vi "llh2lcc.vi"(8 "ecef ref":dbl[](array[numeric]) format="%#_19f", 9 "hgt":dbl, 10 "lon":dbl, 11 "lat":dbl) -> (3 "lcc":dbl[](array[numeric]))   [LabVIEW 2015]
uses:
  <vilib>/Analysis/Matrix/Numeric/Conversions/Array To Matrix - RA.vi
  <vilib>/Analysis/Matrix/Numeric/Conversions/Array To Matrix - RA2.vi
  <vilib>/Analysis/Matrix/Numeric/Multiply/Multiply - RM,RM.vi
  <vilib>/Analysis/Matrix/Numeric/Conversions/Matrix To Array - RM.vi
  <vilib>/Analysis/Matrix/NI_Matrix.lvlib
panel:
  out "ecef":dbl[](array[numeric]) format="%#_19f"
  out "DCM(ecef2lcc)":dbl[][](array[numeric])
  out "N":dbl format="%#_19f"
  out "b^2/a^2":dbl
  out "cos(lam)":dbl
  out "sin(lam)":dbl
  out "sin(phi)":dbl
  out "cos(phi)":dbl
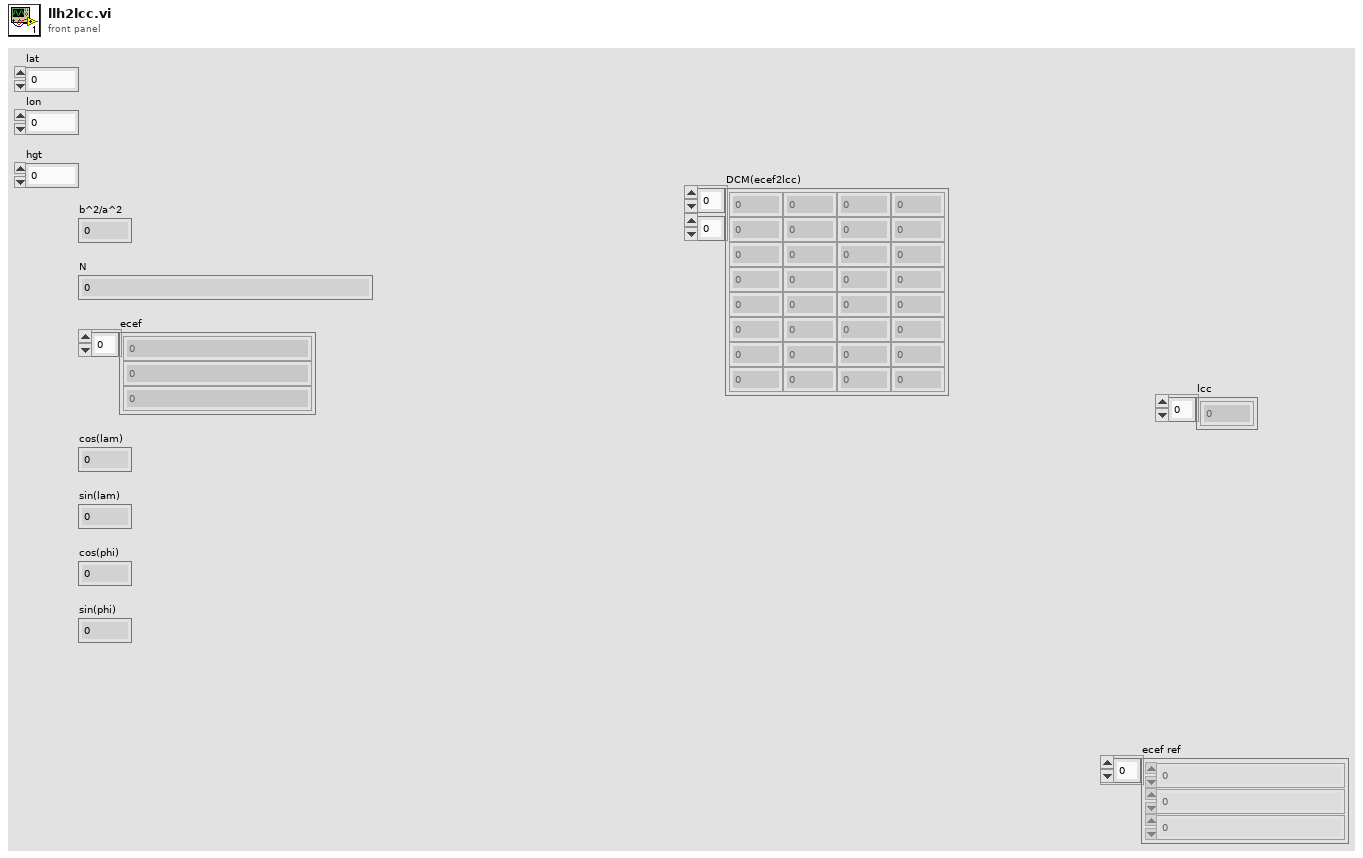
[diagram p1: front panel]
types:
  T1 = typedef "NI_Matrix.lvlib/RealMatrix.ctl" = dbl[][]
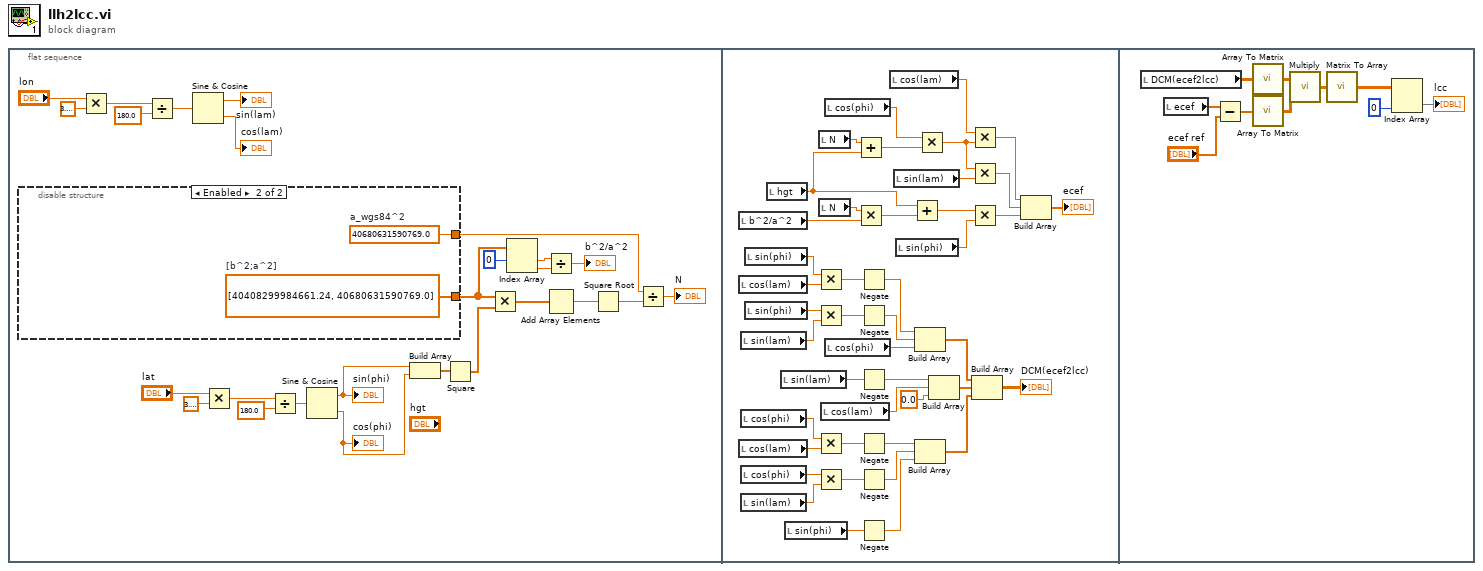
[diagram p0: block diagram]
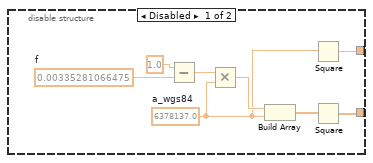
[diagram p2: hidden frame]
diagram:
  n1 = flat-sequence {
    frame #0 {
      n2 = disable-structure shown="Enabled" {
        disable-tunnel: [w29 w36] -> w16
        disable-tunnel: [w27 w35] -> w13
        frame Disabled {
          w34 = 0.00335281066475  # f
          w28 = 6378137.0  # a_wgs84
          n3 = Subtract(x=1.0, y=w34) -> (x-y=w32:dbl)
          n4 = Multiply(x=w32, y=w28) -> (x*y=w31:dbl)
          n5 = Build Array(w31, w28) -> (w30:dbl[])
          n6 = Square(x=w28) -> (x^2=w27:dbl)
          n7 = Square(x=w30) -> (x^2=w29:dbl[])
        }
        frame Enabled {
          w35 = 40680631590769.0  # a_wgs84^2
          w36 = dbl[] [40408299984661.24, 40680631590769.0]  # [b^2;a^2]
        }
      }
      n8 = Multiply(x="lon", y=3.141592653589793) -> (x*y=w23:dbl)
      n9 = Divide(x=w23, y=180.0) -> (x/y=w21:dbl)
      n10 = Sine & Cosine(0:w21) -> (1:→"sin(lam)":dbl, 2:→"cos(lam)":dbl)
      n11 = Multiply(x="lat", y=3.141592653589793) -> (x*y=w4:dbl)
      n12 = Divide(x=w4, y=180.0) -> (x/y=w6:dbl)
      n13 = Sine & Cosine(0:w6) -> (1:w7:dbl, 2:w8:dbl)
      "sin(phi)" <- w7
      "cos(phi)" <- w8
      n14 = Build Array(w7, w8) -> (w9:dbl[])
      n15 = Square(x=w9) -> (x^2=w10:dbl[])
      n16 = Multiply(x=w16, y=w10) -> (x*y=w15:dbl[])
      n17 = Index Array(array=w16, index #1=0 ("index")) -> (element #1=w18:dbl, element #2=w19:dbl)  [unwired: 1 in]
      n18 = Divide(x=w18, y=w19) -> (x/y=→"b^2/a^2":dbl)
      n19 = Add Array Elements(numeric array=w15) -> (sum=w11:dbl)
      n20 = Square Root(x=w11) -> (sqrt(x)=w14:dbl)
      n21 = Divide(x=w13, y=w14) -> (x/y=→"N":dbl)
    }
    frame #1 {
      n22 = local read "b^2/a^2"() -> (w68:dbl)
      n23 = local read "cos(lam)"() -> (w62:dbl)
      n24 = local read "cos(lam)"() -> (w44:dbl)
      n25 = local read "sin(lam)"() -> (w59:dbl)
      n26 = local read "cos(phi)"() -> (w43:dbl)
      n27 = local read "cos(phi)"() -> (w48:dbl)
      n28 = local read "sin(lam)"() -> (w47:dbl)
      n29 = local read "sin(phi)"() -> (w63:dbl)
      n30 = local read "sin(phi)"() -> (w58:dbl)
      n31 = local read "hgt"() -> (w71:dbl)
      n32 = local read "sin(lam)"() -> (w54:dbl)
      n33 = local read "sin(phi)"() -> (w42:dbl)
      n34 = Multiply(x=w63, y=w62) -> (x*y=w61:dbl)
      n35 = Multiply(x=w58, y=w59) -> (x*y=w60:dbl)
      n36 = Multiply(x=w43, y=w44) -> (x*y=w45:dbl)
      n37 = Multiply(x=w48, y=w47) -> (x*y=w46:dbl)
      n38 = local read "N"() -> (w70:dbl)
      n39 = local read "N"() -> (w69:dbl)
      n40 = local read "cos(lam)"() -> (w52:dbl)
      n41 = local read "cos(phi)"() -> (w66:dbl)
      n42 = local read "cos(phi)"() -> (w55:dbl)
      n43 = Add(x=w70, y=w71) -> (x+y=w79:dbl)
      n44 = Multiply(x=w69, y=w68) -> (x*y=w75:dbl)
      n45 = Negate(x=w61) -> (-x=w57:dbl)
      n46 = Negate(x=w60) -> (-x=w56:dbl)
      n47 = Negate(x=w54) -> (-x=w53:dbl)
      n48 = Negate(x=w45) -> (-x=w49:dbl)
      n49 = Negate(x=w46) -> (-x=w50:dbl)
      n50 = Negate(x=w42) -> (-x=w41:dbl)
      n51 = local read "cos(lam)"() -> (w65:dbl)
      n52 = local read "sin(lam)"() -> (w64:dbl)
      n53 = local read "sin(phi)"() -> (w67:dbl)
      n54 = Add(x=w71, y=w75) -> (x+y=w74:dbl)
      n55 = Build Array(w57, w56, w55) -> (w40:dbl[])
      n56 = Build Array(w49, w50, w41) -> (w38:dbl[])
      n57 = Multiply(x=w66, y=w79) -> (x*y=w78:dbl)
      n58 = Build Array(w53, w52, 0.0 ("element")) -> (w39:dbl[])
      n59 = Multiply(x=w65, y=w78) -> (x*y=w77:dbl)
      n60 = Multiply(x=w78, y=w64) -> (x*y=w76:dbl)
      n61 = Multiply(x=w74, y=w67) -> (x*y=w73:dbl)
      n62 = Build Array(w40, w39, w38) -> (→"DCM(ecef2lcc)":dbl[][])
      n63 = Build Array(w77, w76, w73) -> (→"ecef":dbl[])
    }
    frame #2 {
      n64 = local read "DCM(ecef2lcc)"() -> (w88:dbl[][])
      n65 = local read "ecef"() -> (w89:dbl[])
      n66 = Subtract(x=w89, y="ecef ref") -> (x-y=w86:dbl[])
      n67 = call-poly <vilib>:"Array To Matrix.vi"("Real 2D Array"=w88) -> ("Real Matrix"=w87:T1)
      n68 = call-poly <vilib>:"Array To Matrix.vi"("Real 1D Array"=w86) -> ("Real Matrix (Column Vector)"=w85:T1)
      n69 = call-poly <vilib>:"Multiply.vi"("Real Matrix B"=w85, "Real Matrix A"=w87) -> ("A * B"=w84:T1)
      n70 = call-poly <vilib>:"Matrix To Array.vi"("Real Matrix"=w84) -> ("Real 2D Array"=w83:dbl[][])
      n71 = Index Array(array=w83, index (col)=0 ("disabled index (col)")) -> (element=→"lcc":dbl[])  [unwired: 1 in]
    }
  }
